vi "CalcCifferences.vi"(8 "error in (no error)":errorcluster, 10 "y scan signals UDL":dbl[](array[numeric]), 11 "x scan signals UDL":dbl[](array[numeric])) -> (0 "error out":errorcluster, 3 "difference":dbl[](array[numeric]))   [LabVIEW 2010]
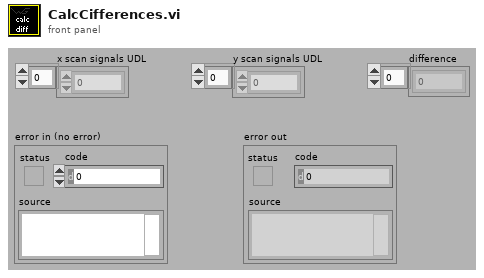
[diagram p1: front panel]
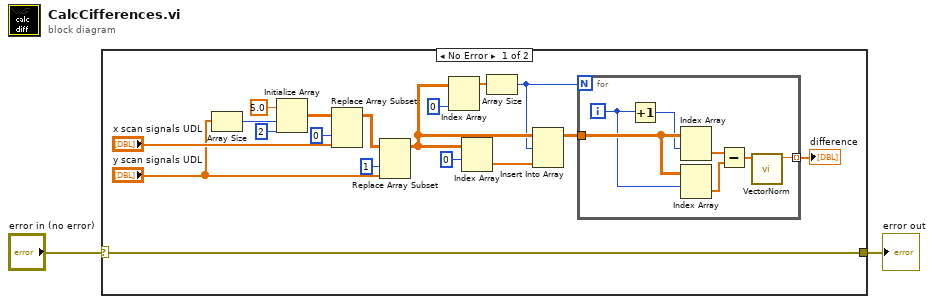
[diagram p0: block diagram]
diagram:
  n1 = case shown="No Error" "error in (no error)" {
    selector: "error in (no error)" -> [w3 w28]
    tunnel: [w3 w28] -> w1
    frame No Error {
      n2 = Array Size(array="y scan signals UDL") -> (size(s)=w5:i32)
      n3 = Initialize Array(5.0 ("element"), w5, 2 ("dimension size")) -> (w11:dbl[][])
      n4 = Replace Array Subset(array=w11, new element="x scan signals UDL", index (col)=0 ("disabled index (col)")) -> (w9:dbl[][])  [unwired: 1 in]
      n5 = Replace Array Subset(array=w9, new element="y scan signals UDL", index (col)=1 ("disabled index (col)")) -> (w7:dbl[][])  [unwired: 1 in]
      n6 = Index Array(array=w7, index (col)=0 ("disabled index (col)")) -> (element=w19:dbl[])  [unwired: 1 in]
      n7 = Index Array(array=w7, index (row)=0) -> (element=w17:dbl[])  [unwired: 1 in]
      n8 = Array Size(array=w19) -> (size(s)=w4:i32)
      n9 = Insert Into Array(array=w7, index (row)=w4, new element=w17) -> (w16:dbl[][])  [unwired: 1 in]
      n10 = for {
        N: w4 -> [_]
        tunnel: w16 -> [w27]
        tunnel: [w21] -> w15 mode=indexing
        i -> [w25]
        n11 = Increment(x=w25) -> (x+1=w26:i32)
        n12 = Index Array(array=w27, index (row)=w26) -> (element=w24:dbl[])  [unwired: 1 in]
        n13 = Index Array(array=w27, index (row)=w25) -> (element=w23:dbl[])  [unwired: 1 in]
        n14 = Subtract(x=w24, y=w23) -> (x-y=w22:dbl[])
        n15 = call "VectorNorm.vi"("Vector"=w22) -> ("Norm"=w21:dbl)  [unwired: 9 in, 1 out]
      }
      "difference" <- w15
    }
    frame Error {
    }
  }
  "error out" <- w1
